vi "rm_duplicated_rows.vi"(1 "Select Data":string[][](array[string])=[["23", "3/22/2019", "30101566", "DM17-20                  ", "                         ", "Fail", "30", "0.14", "1.375", "934.203", "37.774", "0.339"], ["24", "3/22/2019", "30101566", "DM17-20                  ", "                         ", "Fail", "60", "25.11", "1.413", "935.39", "41.68", "29.618"], ["25", "3/22/2019", "30101566", "DM17-20                  ", "                         ", "Fail", "90", "58.98", "1.444", "936.11", "44.048", "45.383"], ["26", "3/22/2019", "30101566", "DM17-20                  ", "                         ", "Fail", "120", "93.3", "1.473", "936.93", "46.745", "52.783"], ["27", "3/22/2019", "30101566", "DM17-20                  ", "                         ", "Fail", "150", "127.7", "1.502", "937.91", "49.969", "56.68"], ["28", "3/22/2019", "30101566", "DM17-20                  ", "                         ", "Fail", "180", "161.8", "1.53", "938.84", "53.028", "58.751"], ["29", "3/22/2019", "30101566", "DM17-20                  ", "                         ", "Fail", "210", "195.3", "1.558", "939.97", "56.745", "59.692"], ["30", "3/22/2019", "30101566", "DM17-20                  ", "                         ", "Fail", "240", "228.2", "1.584", "941.04", "60.265", "60.027"], ["31", "3/22/2019", "30101566", "DM17-20                  ", "                         ", "Fail", "270", "260.1", "1.61", "942.37", "64.64", "59.834"], ["32", "3/22/2019", "30101566", "DM17-20                  ", "                         ", "Fail", "300", "290.9", "1.635", "943.75", "69.18", "59.307"], ["33", "3/22/2019", "30101566", "DM17-20                  ", "                         ", "Fail", "330", "320.2", "1.66", "945.28", "74.212", "58.452"]]) -> (0 "Output Data":string[][](array[string]))   [LabVIEW 2017]
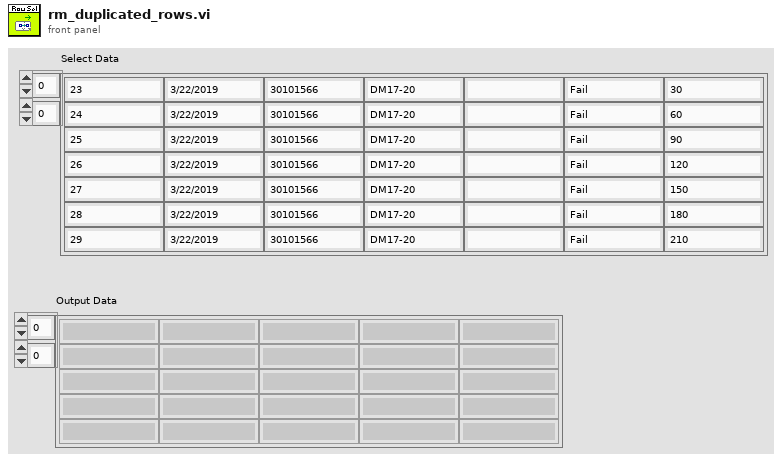
[diagram p1: front panel]
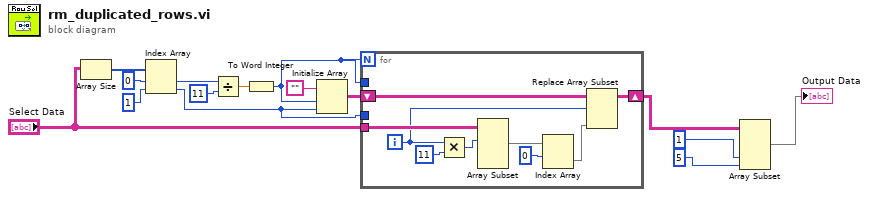
[diagram p0: block diagram]
diagram:
  n1 = Array Size(array="Select Data") -> (size(s)=w15:i32[])
  n2 = Index Array(array=w15, index #1=0 ("index"), index #2=1 ("index")) -> (element #1=w12:i32, element #2=w6:i32)
  n3 = Divide(x=w12, y=11) -> (x/y=w10:dbl)
  n4 = To Word Integer(number=w10) -> (16bit integer=w7:i16)
  n5 = Initialize Array("", w7, w6) -> (w5:string[][])
  n6 = for {
    N: w7 -> [_]
    tunnel: w7 -> [_]
    tunnel: w6 -> [_]
    tunnel: "Select Data" -> [w24]
    shift-right: [w17] -> w4
    shift-left: w5 -> [w19]
    i -> [w16]
    n7 = Multiply(x=w16, y=11) -> (x*y=w22:i32)
    n8 = Array Subset(array=w24, index (row)=w22) -> (w21:string[][])  [unwired: 3 in]
    n9 = Index Array(array=w21, index (row)=0) -> (element=w18:string[])  [unwired: 1 in]
    n10 = Replace Array Subset(array=w19, new element=w18, index (row)=w16) -> (w17:string[][])  [unwired: 1 in]
  }
  n11 = Array Subset(array=w4, index (col)=1 ("length"), length (col)=5 ("index")) -> (→"Output Data":string[][])  [unwired: 2 in]
